vi "test - Tag.vi"(8 "error in (no error)":errorcluster, 11 "TestCase in":refnum<class "testcase-Supported-Datatype.lvclass">) -> (0 "error out":errorcluster, 3 "TestCase out":refnum<class "testcase-Supported-Datatype.lvclass">)   [LabVIEW 2017, in "testcase-Supported-Datatype.lvclass"]
uses:
  testcase-Supported-Datatype.lvclass
  C:/Program Files (x86)/National Instruments/LabVIEW 2017/vi.lib/addons/_JKI Toolkits/VI Tester/TestCase.llb/TestCase.lvclass
  <vilib>/addons/_JKI Toolkits/VI Tester/TestCase.llb/TestCase.lvclass
  4933ebb4-187b-4d02-a477-b811f479a1ff.vi
  0c6b2f80-dfaa-43ae-8da0-6ede34301d28.vi
panel:
  out "data string 2":string
  out "data string":string
  in  "shared variable refnum in":refnum<k21>="ni.var.psp://localhost/System/DAQmx/Server Polling Rate"
  out "shared variable refnum in":refnum<k21>="ni.var.psp://localhost/System/DAQmx/Server Polling Rate"
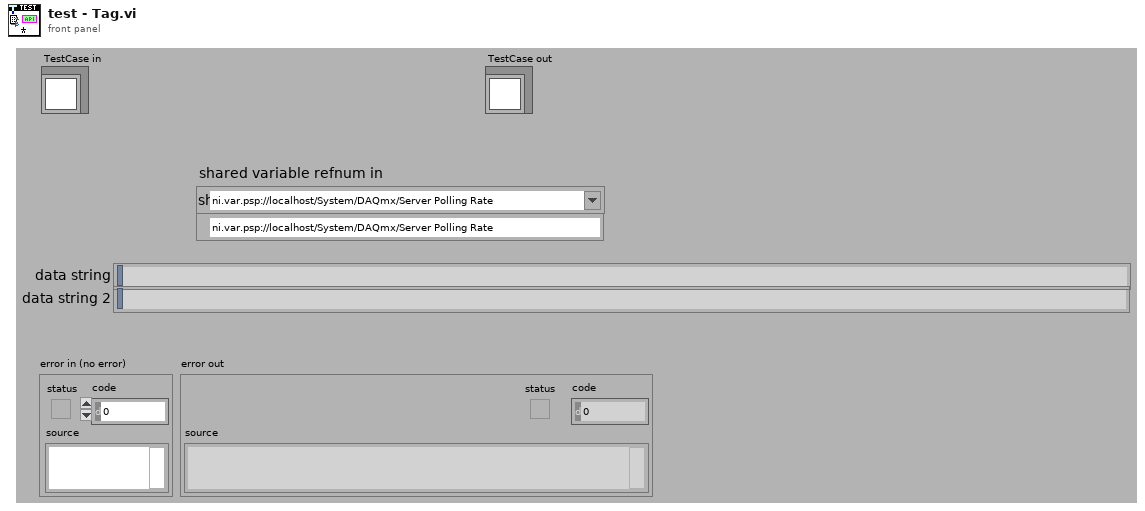
[diagram p1: front panel]
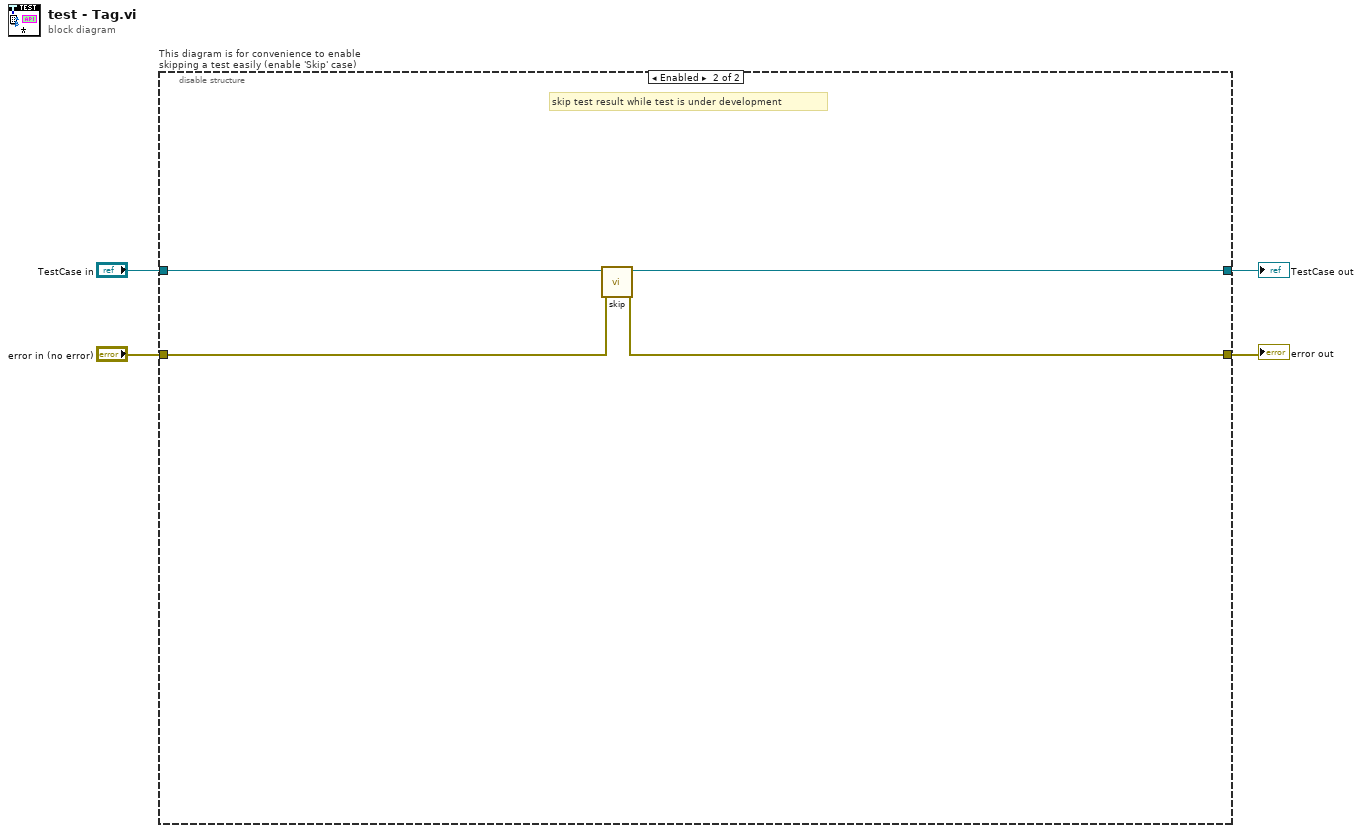
[diagram p0: block diagram]
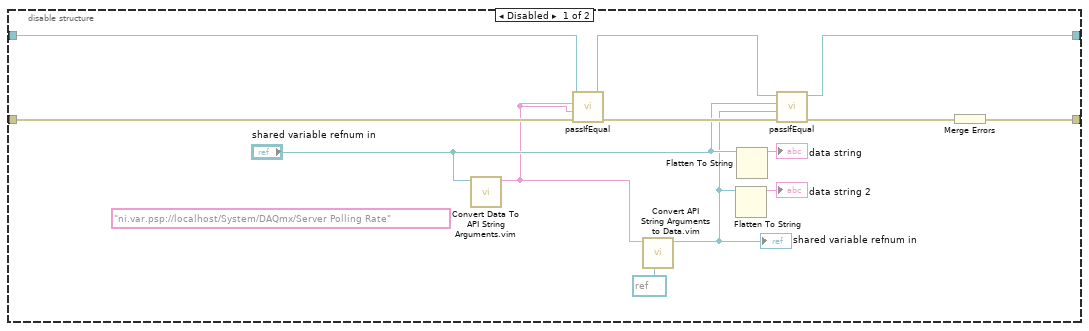
[diagram p2: hidden frame]
diagram:
  n1 = disable-structure "This diagram is for convenience to enable skipping a test easily (enable 'Skip' case)" shown="Enabled" {
    disable-tunnel: "TestCase in" -> [w17 w21]
    disable-tunnel: [w13 w19] -> w1
    disable-tunnel: [w16 w20] -> w3
    disable-tunnel: "error in (no error)" -> [w15 w18]
    frame Disabled {
      (unwired) "ni.var.psp://localhost/System/DAQmx/Server Polling Rate" ("String")
      n2 = call "Convert Data To API String Arguments.vim"("data"="shared variable refnum in") -> ("String"=w5:string)  [unwired: 7 in, 1 out]
      n3 = call-dynamic "passIfEqual.vi"("error in (no error)"=w15, "y"=w5, "x"=w5, "TestCase in"=w17) -> ("error out"=w11:errorcluster, "TestCase out"=w14:refnum<class "testcase-Supported-Datatype.lvclass">)  [unwired: 6 in]
      n4 = call "Convert API String Arguments to Data.vim"("Type"=refnum<k21> refnum ("shared variable refnum in"), "String"=w5) -> ("Data"=w6:refnum<k21>)  [unwired: 6 in, 1 out]
      "shared variable refnum in" <- w6
      n5 = Flatten To String(anything=w6) -> (data string=→"data string 2":string)  [unwired: 3 in, 2 out]
      n6 = Flatten To String(anything="shared variable refnum in") -> (data string=→"data string":string)  [unwired: 3 in, 2 out]
      n7 = call-dynamic "passIfEqual.vi"("error in (no error)"=w11, "y"=w6, "x"="shared variable refnum in", "TestCase in"=w14) -> ("error out"=w12:errorcluster, "TestCase out"=w13:refnum<class "testcase-Supported-Datatype.lvclass">)  [unwired: 6 in]
      n8 = Merge Errors(w12) -> (w16:errorcluster)
    }
    frame Enabled {
      # "skip test result while test is under development"
      n9 = call <vilib>:"skip.vi"("error in (no error)"=w18, "TestCase in"=w21) -> ("error out"=w20:errorcluster, "TestCase out"=w19:refnum<class "testcase-Supported-Datatype.lvclass">)  [unwired: 8 in]
    }
  }
  "error out" <- w3
  "TestCase out" <- w1
